vi "connect to command network stream.vi"(10 "Comms data in":T1={"Parameters"={"error writer name"="error writer", "command reader name"="command reader", "error buffer size"=16, "command buffer size"=16, "scanivalveIP"="", "scanivalvePeriod"=16}, "Variables"={"listen schedule"=0, "incident buffer"=[], "command stream"="", "error stream"="", "waiting for command stream connect"=FALSE, "waiting for error stream connect"=FALSE, "scanivalve connection"=refnum, "scanivalveScheduleID"=16, "activeScanivalvePorts"=[], "channelCount"=0}, "scanivalveConfig"={"listS"={"period"=0, "ADtrig"=FALSE, "ScanTrig"=FALSE, "page"=0, "qpkts"=0}, "listC"={"ZC"=FALSE, "unitScan"="", "CvtUnit"=0.0, "bin"=FALSE, "EU"=FALSE}, "listSG"={"Avg1"=0, "FPS1"=0, "SGEnable1"=FALSE}, "activeChannels"={"Chan1"={"101"=FALSE, "102"=FALSE, "103"=FALSE, "104"=FALSE, "109"=FALSE, "110"=FALSE, "111"=FALSE, "112"=FALSE, "201"=FALSE, "202"=FALSE, "203"=FALSE, "204"=FALSE, "209"=FALSE, "210"=FALSE, "211"=FALSE, "212"=FALSE, "301"=FALSE, "302"=FALSE, "303"=FALSE, "304"=FALSE, "309"=FALSE, "310"=FALSE, "311"=FALSE, "312"=FALSE, "401"=FALSE, "402"=FALSE, "403"=FALSE, "404"=FALSE, "409"=FALSE, "410"=FALSE, "411"=FALSE, "412"=FALSE}}}}, 11 "RT Queues":T8) -> (3 "Comms data out":T1={"Parameters"={"error writer name"="error writer", "command reader name"="command reader", "error buffer size"=16, "command buffer size"=16, "scanivalveIP"="", "scanivalvePeriod"=16}, "Variables"={"listen schedule"=0, "incident buffer"=[], "command stream"="", "error stream"="", "waiting for command stream connect"=FALSE, "waiting for error stream connect"=FALSE, "scanivalve connection"=refnum, "scanivalveScheduleID"=16, "activeScanivalvePorts"=[], "channelCount"=0}, "scanivalveConfig"={"listS"={"period"=0, "ADtrig"=FALSE, "ScanTrig"=FALSE, "page"=0, "qpkts"=0}, "listC"={"ZC"=FALSE, "unitScan"="", "CvtUnit"=0.0, "bin"=FALSE, "EU"=FALSE}, "listSG"={"Avg1"=0, "FPS1"=0, "SGEnable1"=FALSE}, "activeChannels"={"Chan1"={"101"=FALSE, "102"=FALSE, "103"=FALSE, "104"=FALSE, "109"=FALSE, "110"=FALSE, "111"=FALSE, "112"=FALSE, "201"=FALSE, "202"=FALSE, "203"=FALSE, "204"=FALSE, "209"=FALSE, "210"=FALSE, "211"=FALSE, "212"=FALSE, "301"=FALSE, "302"=FALSE, "303"=FALSE, "304"=FALSE, "309"=FALSE, "310"=FALSE, "311"=FALSE, "312"=FALSE, "401"=FALSE, "402"=FALSE, "403"=FALSE, "404"=FALSE, "409"=FALSE, "410"=FALSE, "411"=FALSE, "412"=FALSE}}}})   [LabVIEW 2018]
uses:
  Type Defs/Queues cluster.ctl
  Chris VIs/Message Scheduler/message scheduler.lvclass
  comms data.ctl
  Type Defs/generic incident.ctl
  Github/ICL-LabVIEW_General/Scanivalve API project/full interface/polymorphic/scanivalveConfig.ctl
  Github/ICL-LabVIEW_General/Scanivalve API project/full interface/listS.ctl
  Github/ICL-LabVIEW_General/Scanivalve API project/full interface/listC.ctl
  Github/ICL-LabVIEW_General/Scanivalve API project/full interface/listSG.ctl
  Github/ICL-LabVIEW_General/Scanivalve API project/full interface/chan1.ctl
  Queue VIs/En-queue RT comms element.vi
  <resource>/objmgr/ni.dex.rc
panel:
  out "Is Connected":bool
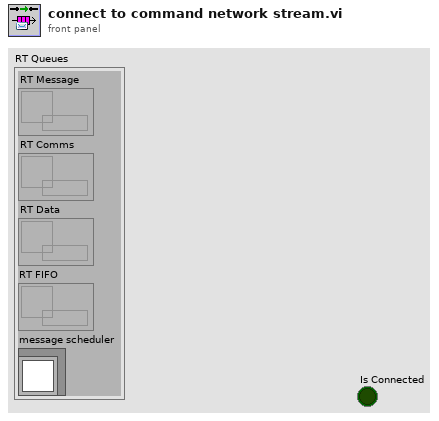
[diagram p1: front panel]
types:
  T1 = typedef "comms data.ctl" = cluster{"Parameters":cluster{"error writer name":string, "command reader name":string, "error buffer size":i32, "command buffer size":i32, "scanivalveIP":string, "scanivalvePeriod":u16}, "Variables":cluster{"listen schedule":u32, "incident buffer":T2[], "command stream":refnum<k21>, "error stream":refnum<k21>, "waiting for command stream connect":bool, "waiting for error stream connect":bool, "scanivalve connection":refnum<k5>, "scanivalveScheduleID":u32, "activeScanivalvePorts":i32[], "channelCount":i16}, "scanivalveConfig":T3}
  T2 = typedef "generic incident.ctl" = cluster{"timestamp":timestamp, "type":string, "Variant":variant}
  T3 = typedef "scanivalveConfig.ctl" = cluster{"listS":T4, "listC":T5, "listSG":T6, "activeChannels":T7}
  T4 = typedef "listS.ctl" = cluster{"period":u16, "ADtrig":bool, "ScanTrig":bool, "page":u16, "qpkts":u16}
  T5 = typedef "listC.ctl" = cluster{"ZC":bool, "unitScan":string, "CvtUnit":dbl, "bin":bool, "EU":bool}
  T6 = typedef "listSG.ctl" = cluster{"Avg1":u16, "FPS1":u16, "SGEnable1":bool}
  T7 = typedef "chan1.ctl" = cluster{"Chan1":cluster{"101":bool, "102":bool, "103":bool, "104":bool, "109":bool, "110":bool, "111":bool, "112":bool, "201":bool, "202":bool, "203":bool, "204":bool, "209":bool, "210":bool, "211":bool, "212":bool, "301":bool, "302":bool, "303":bool, "304":bool, "309":bool, "310":bool, "311":bool, "312":bool, "401":bool, "402":bool, "403":bool, "404":bool, "409":bool, "410":bool, "411":bool, "412":bool}}
  T8 = typedef "Queues cluster.ctl" = cluster{"RT Message":refnum<queue>, "RT Comms":refnum<queue>, "RT Data":refnum<queue>, "RT FIFO":refnum<queue>, "message scheduler":refnum<class "message scheduler.lvclass">}
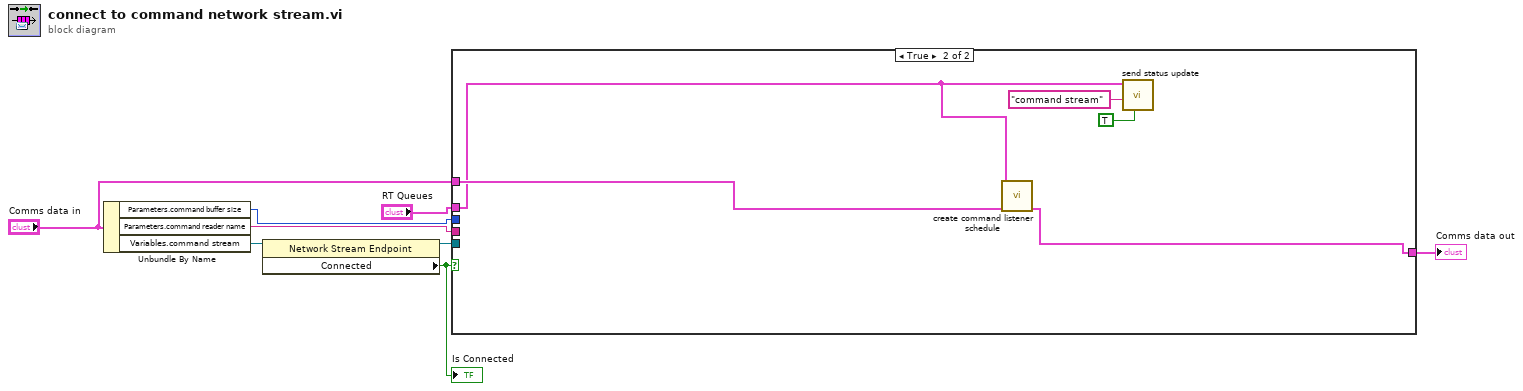
[diagram p0: block diagram]
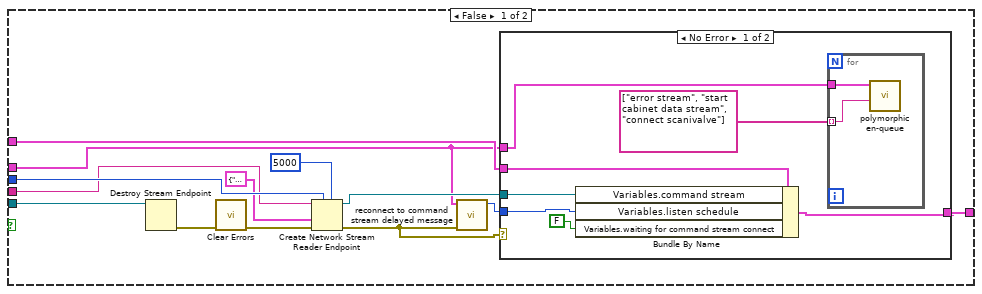
[diagram p2: hidden frame]
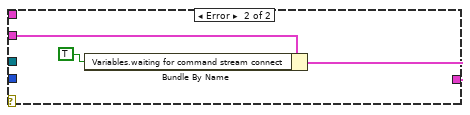
[diagram p3: hidden frame]
diagram:
  n1 = Unbundle By Name("Comms data in") -> ("Parameters.command buffer size"=w5:i32, "Parameters.command reader name"=w4:string, "Variables.command stream"=w8:refnum<k21>)
  n2 = property class="Network Stream Endpoint"(reference=w8) -> (reference out=w3:refnum<k21>, "Connected"=w2:bool)  [unwired: 1 in, 1 out]
  "Is Connected" <- w2
  n3 = case shown="True" w2 {
    tunnel: [w17 w36] -> w7
    tunnel: "Comms data in" -> [w16 w35]
    tunnel: w5 -> [w15 _]
    tunnel: w4 -> [w14 _]
    tunnel: w3 -> [w12 _]
    tunnel: "RT Queues" -> [w9 w34]
    frame False {
      n4 = Destroy Stream Endpoint(11:w12) -> (0:w21:errorcluster)  [unwired: 1 in]
      n5 = call <vilib>:"Clear Errors.vi"("error in (no error)"=w21) -> ("error out"=w11:errorcluster)  [unwired: 5 in, 1 out]
      n6 = Create Network Stream Reader Endpoint(5:5000 ("timeout in ms (-1)"), 7:w15, 8:w11, 9:cluster{"message":string, "data":variant} {"message"="", "data"=variant}, 11:w14) -> (0:w10:errorcluster, 3:w20:refnum<k21>)  [unwired: 2 in]
      n7 = call "reconnect to command stream delayed message.vi"("error in (no error)"=w10, "RT Queues"=w9) -> ("schedule ID"=w19:u32)  [unwired: 9 in]
      n8 = case shown="No Error" w10 {
        tunnel: w20 -> [w28 _]
        tunnel: w19 -> [w25 _]
        tunnel: [w27 w32] -> w17
        tunnel: w16 -> [w26 w33]
        tunnel: w9 -> [w22 _]
        frame No Error {
          n9 = Bundle By Name(cluster=w26, "Variables.command stream"=w28, "Variables.listen schedule"=w25, "Variables.waiting for command stream connect"=FALSE) -> (w27:T1)
          n10 = for {
            tunnel: w22 -> [w30]
            tunnel: string[] ["error stream", "start cabinet data stream", "connect scanivalve"] ("Message") -> [w29] mode=indexing
            n11 = call-poly "polymorphic en-queue.vi"("Message"=w29, "RT Queues"=w30) -> ()  [unwired: 9 in, 1 out]
          }
        }
        frame Error {
          n12 = Bundle By Name(cluster=w33, "Variables.waiting for command stream connect"=TRUE) -> (w32:T1)
        }
      }
    }
    frame True {
      n13 = call "create command listener schedule.vi"("Comms data in"=w35, "RT Queues"=w34) -> ("Comms data out"=w36:T1)  [unwired: 9 in]
      n14 = call "send status update.vi"("status (F)"=TRUE, "subject"="command stream" ("Message"), "RT Queues"=w34) -> ()  [unwired: 8 in, 1 out]
    }
  }
  "Comms data out" <- w7
